vi "FGV_FILE_PATH.vi"(9 "Data In":T2, 11 "Function":enum16{"GET", "SET"}(ring)) -> (1 "Data Out":T1)   [LabVIEW 2015]
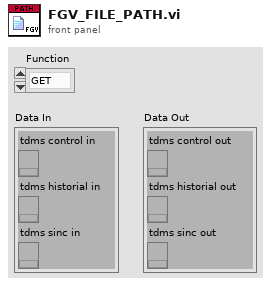
[diagram p1: front panel]
types:
  T1 = cluster{"tdms control out":refnum<k34>, "tdms historial out":refnum<k34>, "tdms sinc out":refnum<k34>}
  T2 = cluster{"tdms control in":refnum<k34>, "tdms historial in":refnum<k34>, "tdms sinc in":refnum<k34>}
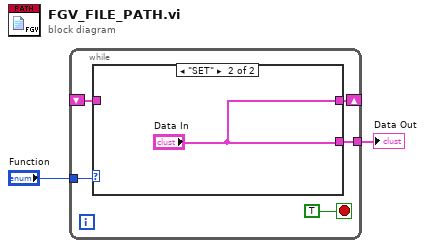
[diagram p0: block diagram]
diagram:
  n1 = while {
    tunnel: "Function" -> [w6]
    shift-right: [w4] -> _
    shift-left: _ -> [w5]
    tunnel: [w3] -> w1
    stop <- TRUE stop-if-true
    n2 = case shown="\"SET\"" w6 {
      tunnel: w5 -> [w8 _]
      tunnel: [w8 "Data In"] -> w4
      tunnel: [w8 "Data In"] -> w3
      frame "GET", Default {
      }
      frame "SET" {
      }
    }
  }
  "Data Out" <- w1
